vi "ServerSide.vi"() -> ()   [LabVIEW 2019]
panel:
  in  "Full Name":string
  in  "Age":dbl
  out "Data  written":i32
  in  "stop Server Side":bool
  in  "Msg":string
  out "connection ID out":refnum<k5>
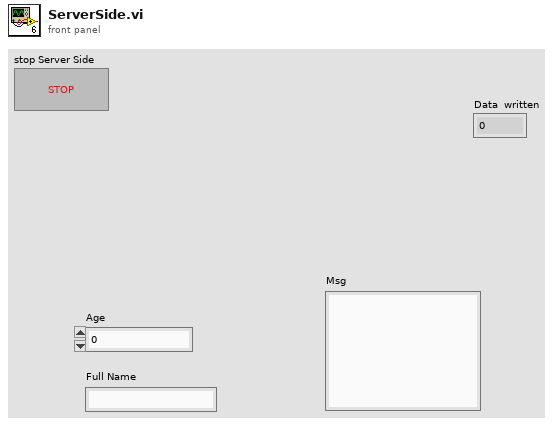
[diagram p1: front panel]
types:
  T1 = cluster{"Age ":dbl, "Full Name":string, "Msg":string}
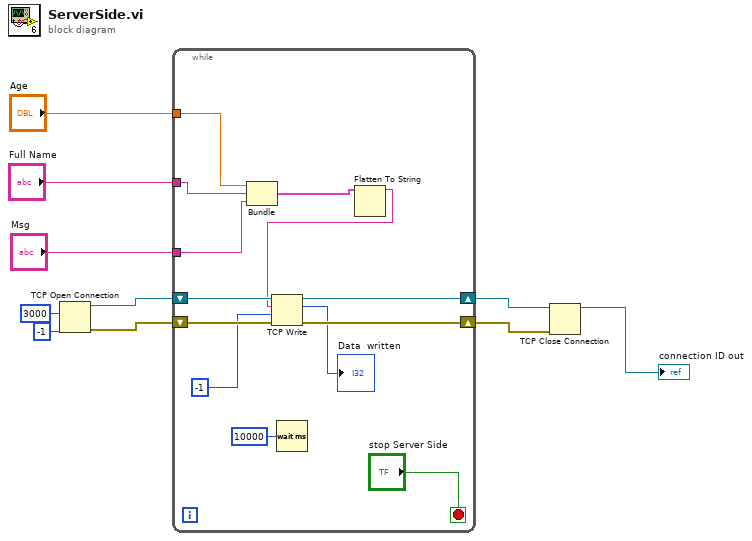
[diagram p0: block diagram]
diagram:
  n1 = TCP Open Connection(remote port or service name=u16 3000, timeout ms (60000)=-1) -> (connection ID=w8:refnum<k5>, error out=w6:errorcluster)  [unwired: 3 in]
  n2 = while {
    shift-right: [w22] -> w7
    shift-left: w8 -> [w23]
    shift-right: [w20] -> w5
    shift-left: w6 -> [w21]
    tunnel: "Age" -> [w15]
    tunnel: "Full Name" -> [w14]
    tunnel: "Msg" -> [w13]
    stop <- "stop Server Side" stop-if-true
    n3 = Bundle "Bundle"("Age"=w15, "Full Name"=w14, "Msg"=w13) -> (w12:T1)  [unwired: 1 in]
    n4 = Wait (ms)(milliseconds to wait=u32 10000) -> ()  [unwired: 1 out]
    n5 = Flatten To String(anything=w12) -> (data string=w11:string)  [unwired: 3 in, 2 out]
    n6 = TCP Write(connection ID=w23, data in=w11, error in (no error)=w21, 9:-1 ("timeout ms (25000)")) -> (connection ID out=w22:refnum<k5>, bytes written=→"Data  written":i32, error out=w20:errorcluster)
  }
  n7 = TCP Close Connection(connection ID=w7, error in (no error)=w5) -> (connection ID out=→"connection ID out":refnum<k5>)  [unwired: 1 in, 1 out]
